vi "TestSTuffs.vi"(8 "error in":errorcluster, 9 "RobotType":T9, 11 "UART port in":T13) -> (2 "iRobot SensorGroup6":T10={"Bumps + Wheel Drops"={"Wheeldrop Caster"=FALSE, "Wheeldrop Left"=FALSE, "Wheeldrop Right"=FALSE, "Bump Left"=FALSE, "Bump Right"=FALSE}, "Wall"=FALSE, "Cliff Left"=FALSE, "Cliff Front Left"=FALSE, "Cliff Front Right"=FALSE, "Cliff Right"=FALSE, "Wall Signal"=0, "Cliff Left Signal"=0, "Cliff Front Left Signal"=0, "Cliff Front Right Signal"=0, "Cliff Right Signal"=0, "Buttons"={"Advance"=FALSE, "Play"=FALSE}, "Virtual Wall"=FALSE, "# Stream Packets"=0, "Requested Velocity (mm/s)"=0, "Requested Radius (mm)"=0, "Requested Right Wheel Velocity (mm/s)"=0, "Requested Left Wheel Velocity (mm/s)"=0, "Distance (mm)"=0, "Angle (deg)"=0, "Song Playing"=FALSE, "Song Number"=0, "Charging State"=enum."Not Charging", "Voltage (mV)"=0, "Current (mA)"=0, "Battery Temperature (deg C)"=0, "Battery Charge (mAh)"=0, "Battery Capacity (mAh)"=0, "Charging Sources"={"Internal Charger"=FALSE, "Home Base"=FALSE}, "OI Mode"=enum."Off", "Digital Inputs"={"Digital Input 0"=FALSE, "Digital Input 1"=FALSE, "Digital Input 2"=FALSE, "Digital Input 3"=FALSE, "Device Detect"=FALSE}, "Drivers & Wheel Overcurrent"={"Low-Side Driver 0"=FALSE, "Low-Side Driver 1"=FALSE, "Low-Side Driver 2"=FALSE, "Left Wheel"=FALSE, "Right Wheel"=FALSE}, "Analog Signal"=0, "Infrared"=255} {"Infrared" format="%02x"}, 3 "UART port out":T13, 4 "Kobuki Sensors  out":T1={"Bumps + Wheel Drops"={"Wheeldrop Left"=FALSE, "Wheeldrop Right"=FALSE, "Bump Left"=FALSE, "Bump Center"=FALSE, "Bump Right"=FALSE}, "Cliff Left"=FALSE, "Cliff Center"=FALSE, "Cliff Right"=FALSE, "Cliff Left Signal"=0, "Cliff Center Signal"=0, "Cliff Right Signal"=0, "Buttons"={"B0"=FALSE, "B1"=FALSE, "B2"=FALSE}, "# Stream Packets"=0, "Requested Velocity (mm/s)"=0, "Requested Radius (mm)"=0, "Requested Right Wheel Velocity (mm/s)"=0, "Requested Left Wheel Velocity (mm/s)"=0, "Left Wheel Encoder (ticks)"=0, "Angle (deg)"=0, "Song Playing"=FALSE, "Song Number"=0, "Charging State"=enum."Not Charging", "Voltage (mV)"=0, "Current (mA)"=0, "Battery Temperature (deg C)"=0, "Battery Charge (mAh)"=0, "Battery Capacity (mAh)"=0, "Charging Sources"={"Internal Charger"=FALSE, "Home Base"=FALSE}, "OI Mode"=enum."Off", "Digital Inputs"={"Digital Input 0"=FALSE, "Digital Input 1"=FALSE, "Digital Input 2"=FALSE, "Digital Input 3"=FALSE, "Device Detect"=FALSE}, "Drivers & Wheel Overcurrent"={"Low-Side Driver 0"=FALSE, "Low-Side Driver 1"=FALSE, "Low-Side Driver 2"=FALSE, "Left Wheel"=FALSE, "Right Wheel"=FALSE}, "Analog Signal"=0, "Infrared"=255, "Right Wheel Encoder (ticks) "=0, "TimeStamp"=0} {"Infrared" format="%02x"}, 5 "net angle (deg)":i32, 7 "net distance (mm)":i32)   [LabVIEW 2014]
uses:
  iRobot/Advanced/UART/iRobot UART Port Type.ctl
  iRobot/Sensor/Sensor Group 6.ctl
  iRobot/Sensor/Bumps + Wheel Drops.ctl
  iRobot/Sensor/Buttons.ctl
  iRobot/Sensor/Charging State.ctl
  iRobot/Sensor/Charging Sources Available.ctl
  iRobot/Sensor/OI Mode.ctl
  iRobot/Sensor/Cargo Bay Digital Inputs.ctl
  iRobot/Sensor/Low-Side Driver + Wheel Overcurrent.ctl
  RobotType.ctl
  Kobuki/KobukiSensors.ctl
  Kobuki/Kobuki Bumps and WheelDrops.ctl
  Kobuki/Kobuki Buttons.ctl
panel:
  out "NetAngle":dbl
  out "NetDistance":dbl
  out "Accumulator":i16
  out "Accumulator 2":i16
  in  "ResetOdo":bool
  in  "Left Wheel Encoder (ticks)":i16
  in  "Right Wheel Encoder (ticks)":i16 format="%.0x"
  in  "Stop Button":bool
  in  "Kobuki Sensors  out 2":T1={"Bumps + Wheel Drops"={"Wheeldrop Left"=FALSE, "Wheeldrop Right"=FALSE, "Bump Left"=FALSE, "Bump Center"=FALSE, "Bump Right"=FALSE}, "Cliff Left"=FALSE, "Cliff Center"=FALSE, "Cliff Right"=FALSE, "Cliff Left Signal"=0, "Cliff Center Signal"=0, "Cliff Right Signal"=0, "Buttons"={"B0"=FALSE, "B1"=FALSE, "B2"=FALSE}, "# Stream Packets"=0, "Requested Velocity (mm/s)"=0, "Requested Radius (mm)"=0, "Requested Right Wheel Velocity (mm/s)"=0, "Requested Left Wheel Velocity (mm/s)"=0, "Left Wheel Encoder (ticks)"=0, "Angle (deg)"=0, "Song Playing"=FALSE, "Song Number"=0, "Charging State"=enum."Not Charging", "Voltage (mV)"=0, "Current (mA)"=0, "Battery Temperature (deg C)"=0, "Battery Charge (mAh)"=0, "Battery Capacity (mAh)"=0, "Charging Sources"={"Internal Charger"=FALSE, "Home Base"=FALSE}, "OI Mode"=enum."Off", "Digital Inputs"={"Digital Input 0"=FALSE, "Digital Input 1"=FALSE, "Digital Input 2"=FALSE, "Digital Input 3"=FALSE, "Device Detect"=FALSE}, "Drivers & Wheel Overcurrent"={"Low-Side Driver 0"=FALSE, "Low-Side Driver 1"=FALSE, "Low-Side Driver 2"=FALSE, "Left Wheel"=FALSE, "Right Wheel"=FALSE}, "Analog Signal"=0, "Infrared"=255, "Right Wheel Encoder (ticks) "=0, "TimeStamp"=0} {"Infrared" format="%02x"}
  # "Electrical: charging, battery, OI mode"
  # "Sensors: bump, cliff, button, wheel drop, wall, virtual wall"
  # "Motion: distance, angle, requested velocity"
  # "Cargo Bay: I/O, overcurrent, infrared"
  # "Song"
  # "Electrical: charging, battery, OI mode"
  # "Sensors: bump, cliff, button, wheel drop, wall, virtual wall"
  # "Motion: distance, angle, requested velocity"
  # "Cargo Bay: I/O, overcurrent, infrared"
  # "Song"
  # "Electrical: charging, battery, OI mode"
  # "Sensors: bump, cliff, button, wheel drop, wall, virtual wall"
  # "Motion: distance, angle, requested velocity"
  # "Cargo Bay: I/O, overcurrent, infrared"
  # "Song"
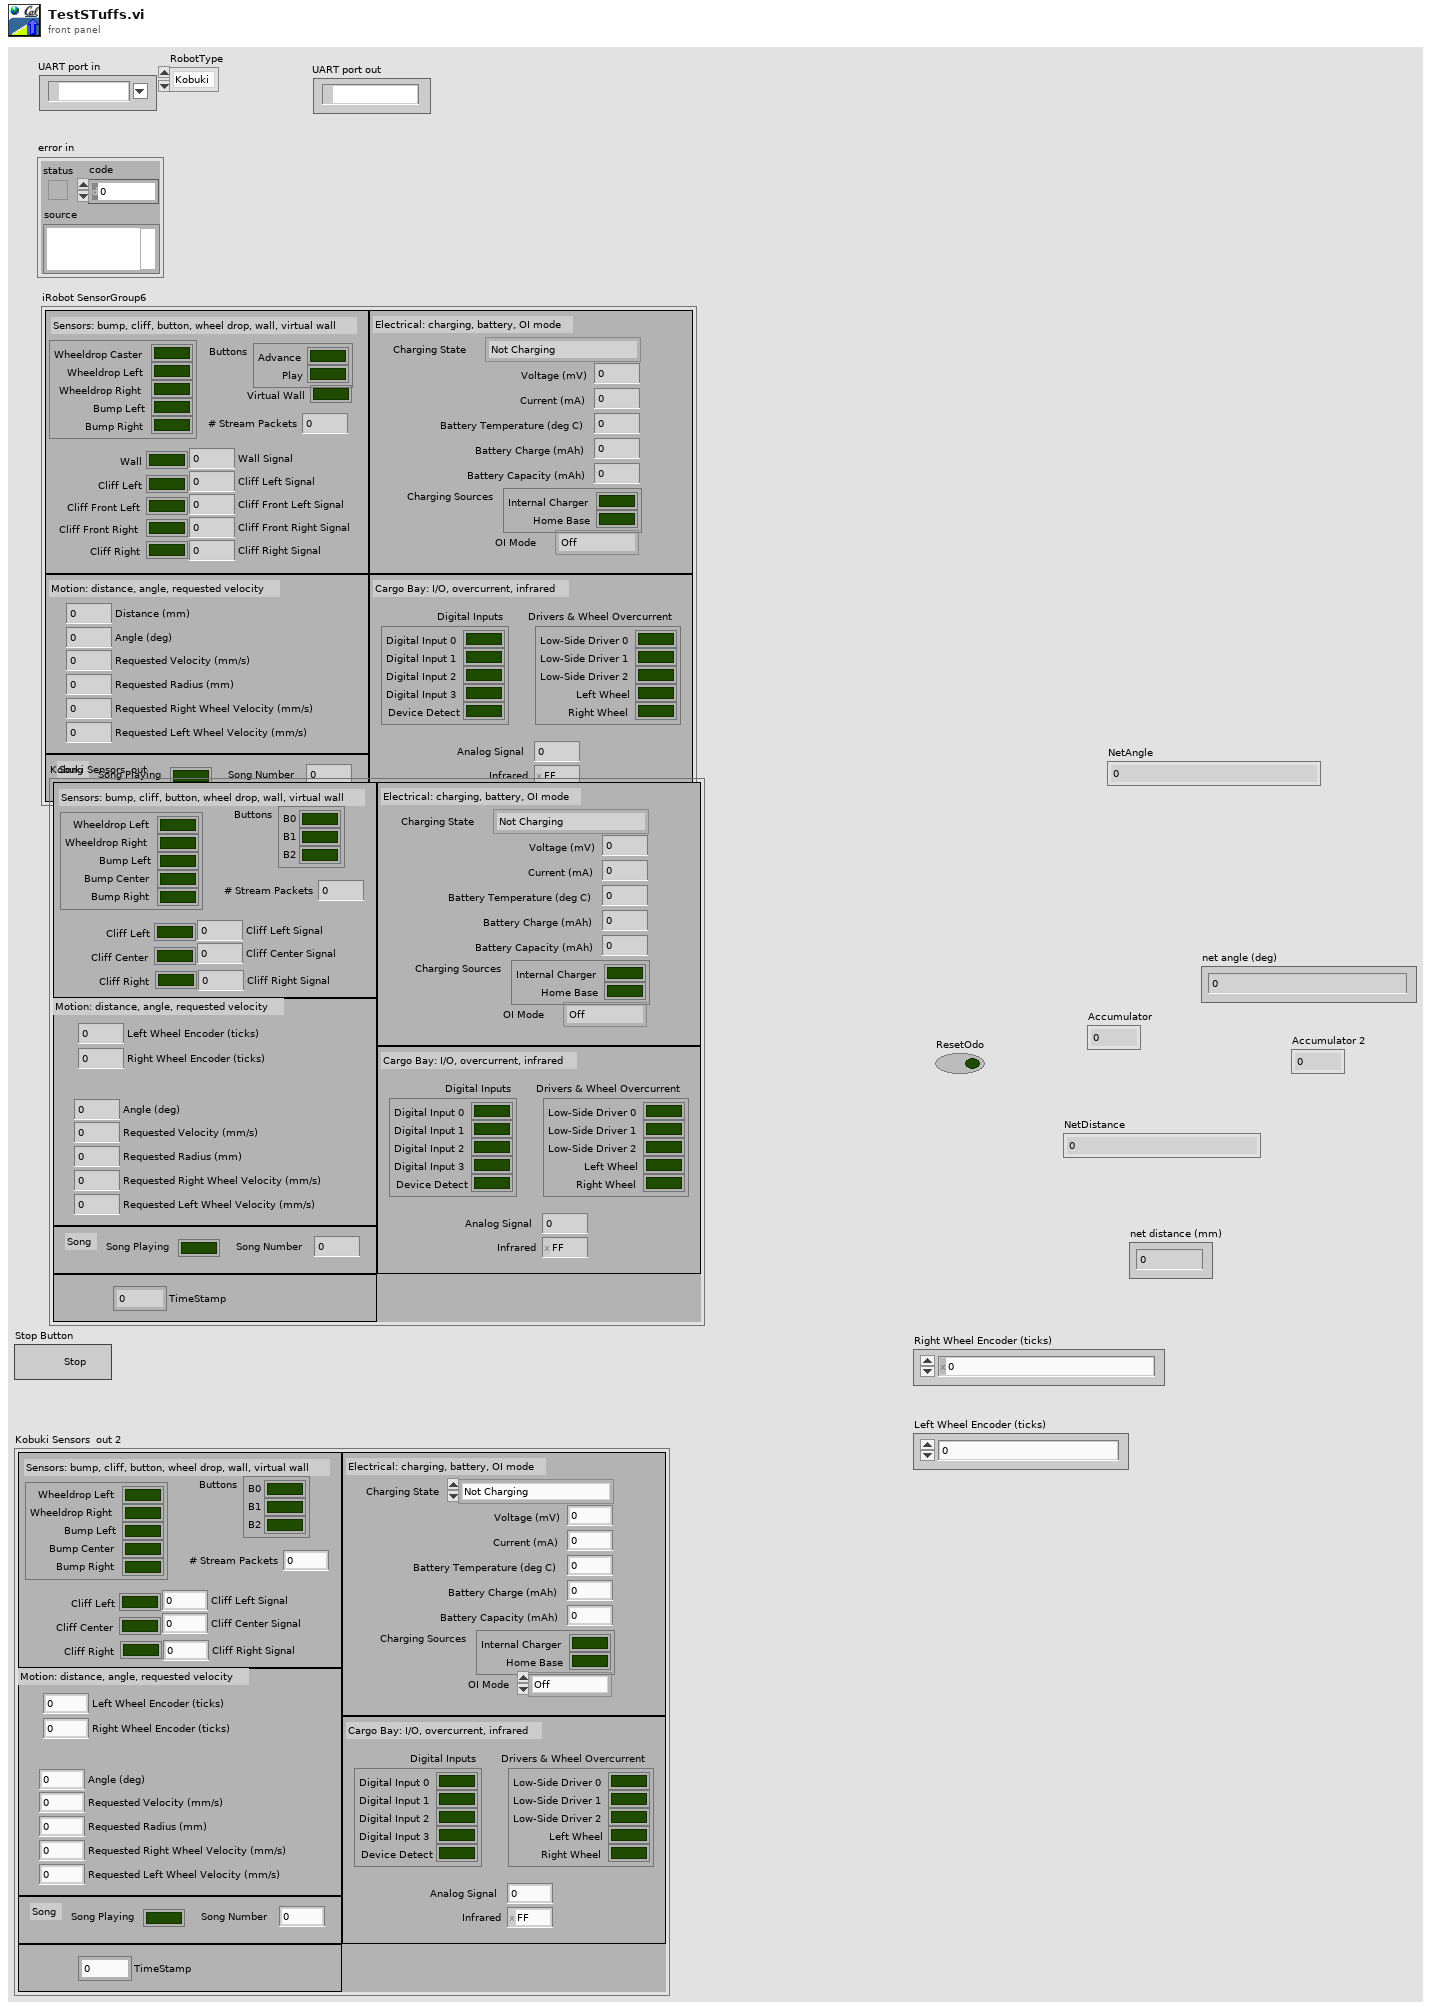
[diagram p1: front panel]
types:
  T1 = typedef "KobukiSensors.ctl" = cluster{"Bumps + Wheel Drops":T2, "Cliff Left":bool, "Cliff Center":bool, "Cliff Right":bool, "Cliff Left Signal":u16, "Cliff Center Signal":u16, "Cliff Right Signal":u16, "Buttons":T3, "# Stream Packets":u8, "Requested Velocity (mm/s)":i16, "Requested Radius (mm)":i16, "Requested Right Wheel Velocity (mm/s)":i16, "Requested Left Wheel Velocity (mm/s)":i16, "Left Wheel Encoder (ticks)":i16, "Angle (deg)":i32, "Song Playing":bool, "Song Number":u8, "Charging State":T4, "Voltage (mV)":u16, "Current (mA)":i16, "Battery Temperature (deg C)":i8, "Battery Charge (mAh)":u16, "Battery Capacity (mAh)":u16, "Charging Sources":T5, "OI Mode":T6, "Digital Inputs":T7, "Drivers & Wheel Overcurrent":T8, "Analog Signal":u16, "Infrared":u8, "Right Wheel Encoder (ticks) ":i16, "TimeStamp":u16}
  T2 = typedef "Kobuki Bumps and WheelDrops.ctl" = cluster{"Wheeldrop Left":bool, "Wheeldrop Right":bool, "Bump Left":bool, "Bump Center":bool, "Bump Right":bool}
  T3 = typedef "Kobuki Buttons.ctl" = cluster{"B0":bool, "B1":bool, "B2":bool}
  T4 = typedef "Charging State.ctl" = enum16{"Not Charging", "Reconditioning Charging", "Full Charging", "Trickle Charging", "Waiting", "Charging Fault Condition"}
  T5 = typedef "Charging Sources Available.ctl" = cluster{"Internal Charger":bool, "Home Base":bool}
  T6 = typedef "OI Mode.ctl" = enum16{"Off", "Passive", "Safe", "Full"}
  T7 = typedef "Cargo Bay Digital Inputs.ctl" = cluster{"Digital Input 0":bool, "Digital Input 1":bool, "Digital Input 2":bool, "Digital Input 3":bool, "Device Detect":bool}
  T8 = typedef "Low-Side Driver + Wheel Overcurrent.ctl" = cluster{"Low-Side Driver 0":bool, "Low-Side Driver 1":bool, "Low-Side Driver 2":bool, "Left Wheel":bool, "Right Wheel":bool}
  T9 = typedef "RobotType.ctl" = enum16{"Kobuki", "iRobot"}
  T10 = typedef "Sensor Group 6.ctl" = cluster{"Bumps + Wheel Drops":T11, "Wall":bool, "Cliff Left":bool, "Cliff Front Left":bool, "Cliff Front Right":bool, "Cliff Right":bool, "Wall Signal":u16, "Cliff Left Signal":u16, "Cliff Front Left Signal":u16, "Cliff Front Right Signal":u16, "Cliff Right Signal":u16, "Buttons":T12, "Virtual Wall":bool, "# Stream Packets":u8, "Requested Velocity (mm/s)":i16, "Requested Radius (mm)":i16, "Requested Right Wheel Velocity (mm/s)":i16, "Requested Left Wheel Velocity (mm/s)":i16, "Distance (mm)":i32, "Angle (deg)":i32, "Song Playing":bool, "Song Number":u8, "Charging State":T4, "Voltage (mV)":u16, "Current (mA)":i16, "Battery Temperature (deg C)":i8, "Battery Charge (mAh)":u16, "Battery Capacity (mAh)":u16, "Charging Sources":T5, "OI Mode":T6, "Digital Inputs":T7, "Drivers & Wheel Overcurrent":T8, "Analog Signal":u16, "Infrared":u8}
  T11 = typedef "Bumps + Wheel Drops.ctl" = cluster{"Wheeldrop Caster":bool, "Wheeldrop Left":bool, "Wheeldrop Right":bool, "Bump Left":bool, "Bump Right":bool}
  T12 = typedef "Buttons.ctl" = cluster{"Advance":bool, "Play":bool}
  T13 = typedef "iRobot UART Port Type.ctl" = refnum<visa-resource-name>
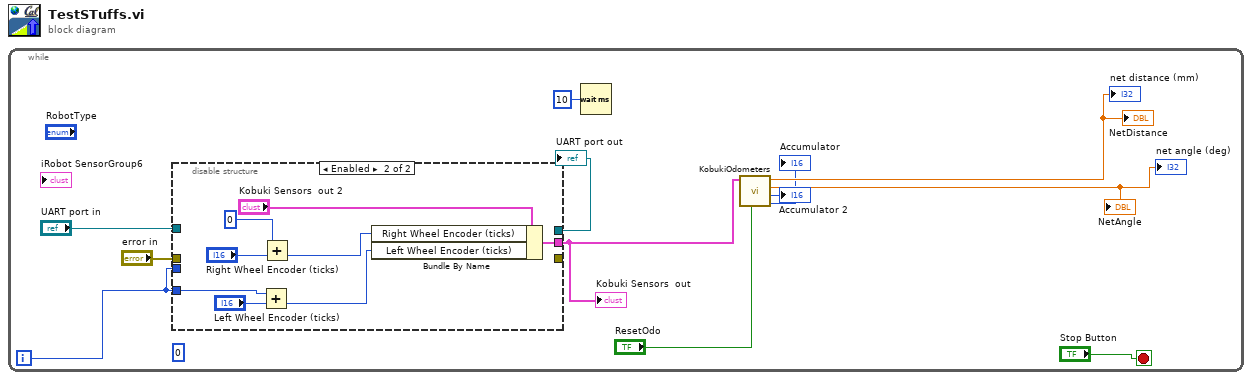
[diagram p0: block diagram]
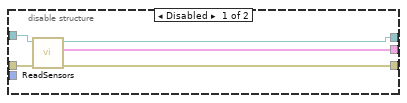
[diagram p2: hidden frame]
diagram:
  n1 = while {
    i -> [w4]
    stop <- "Stop Button" stop-if-true
    (unwired) i64 0 ("y")
    n2 = disable-structure shown="Enabled" {
      disable-tunnel: "UART port in" -> [w17 _]
      disable-tunnel: "error in" -> [w16 _]
      disable-tunnel: [w15 _] -> _
      disable-tunnel: [w14 _] -> w8
      disable-tunnel: [w13 w24] -> w7
      disable-tunnel: w4 -> [_ w20]
      disable-tunnel: w4 -> [_ _]
      frame Disabled {
        n3 = call "ReadSensors.vi"("error in"=w16, "UART in"=w17) -> ("error out"=w15:errorcluster, "Kobuki Sensors  out"=w13:T1, "UART out"=w14:refnum<visa-resource-name>)  [unwired: 7 in]
      }
      frame Enabled {
        n4 = Add(x=w20, y="Left Wheel Encoder (ticks)") -> (x+y=w21:i32)
        n5 = Add(x=i16 0, y="Right Wheel Encoder (ticks)") -> (x+y=w19:i16)
        n6 = Bundle By Name(cluster="Kobuki Sensors  out 2", "Right Wheel Encoder (ticks)"=w19, "Left Wheel Encoder (ticks)"=w21) -> (w24:T1)
      }
    }
    "UART port out" <- w8
    "Kobuki Sensors  out" <- w7
    n7 = Wait (ms)(milliseconds to wait=u32 10) -> ()  [unwired: 1 out]
    n8 = call "KobukiOdometers.vi"("ResetOdo"="ResetOdo", "Kobuki Sensors  in"=w7) -> ("Accumulator"=→"Accumulator":i16, "Accumulator 2"=→"Accumulator 2":i16, "NetAngle"=→"net angle (deg)" →"NetAngle":dbl, "NetDistance"=→"net distance (mm)" →"NetDistance":dbl)  [unwired: 6 in]
  }
